vi "0516205_鍾禾翊_HW2.vi"() -> ()   [LabVIEW 2018]
panel:
  out "ByNum":dbl[](array[numeric])
  out "ByNum":dbl
  out "Slope":bool
  out "size(s)":i32[](array[numeric])
  out "Result Array":dbl[][](array[numeric])
  in  "Input N":i32=4
  out "Array 3":i32[](array[numeric])
  # "By 0"
  # "By 1"
  # "By 2"
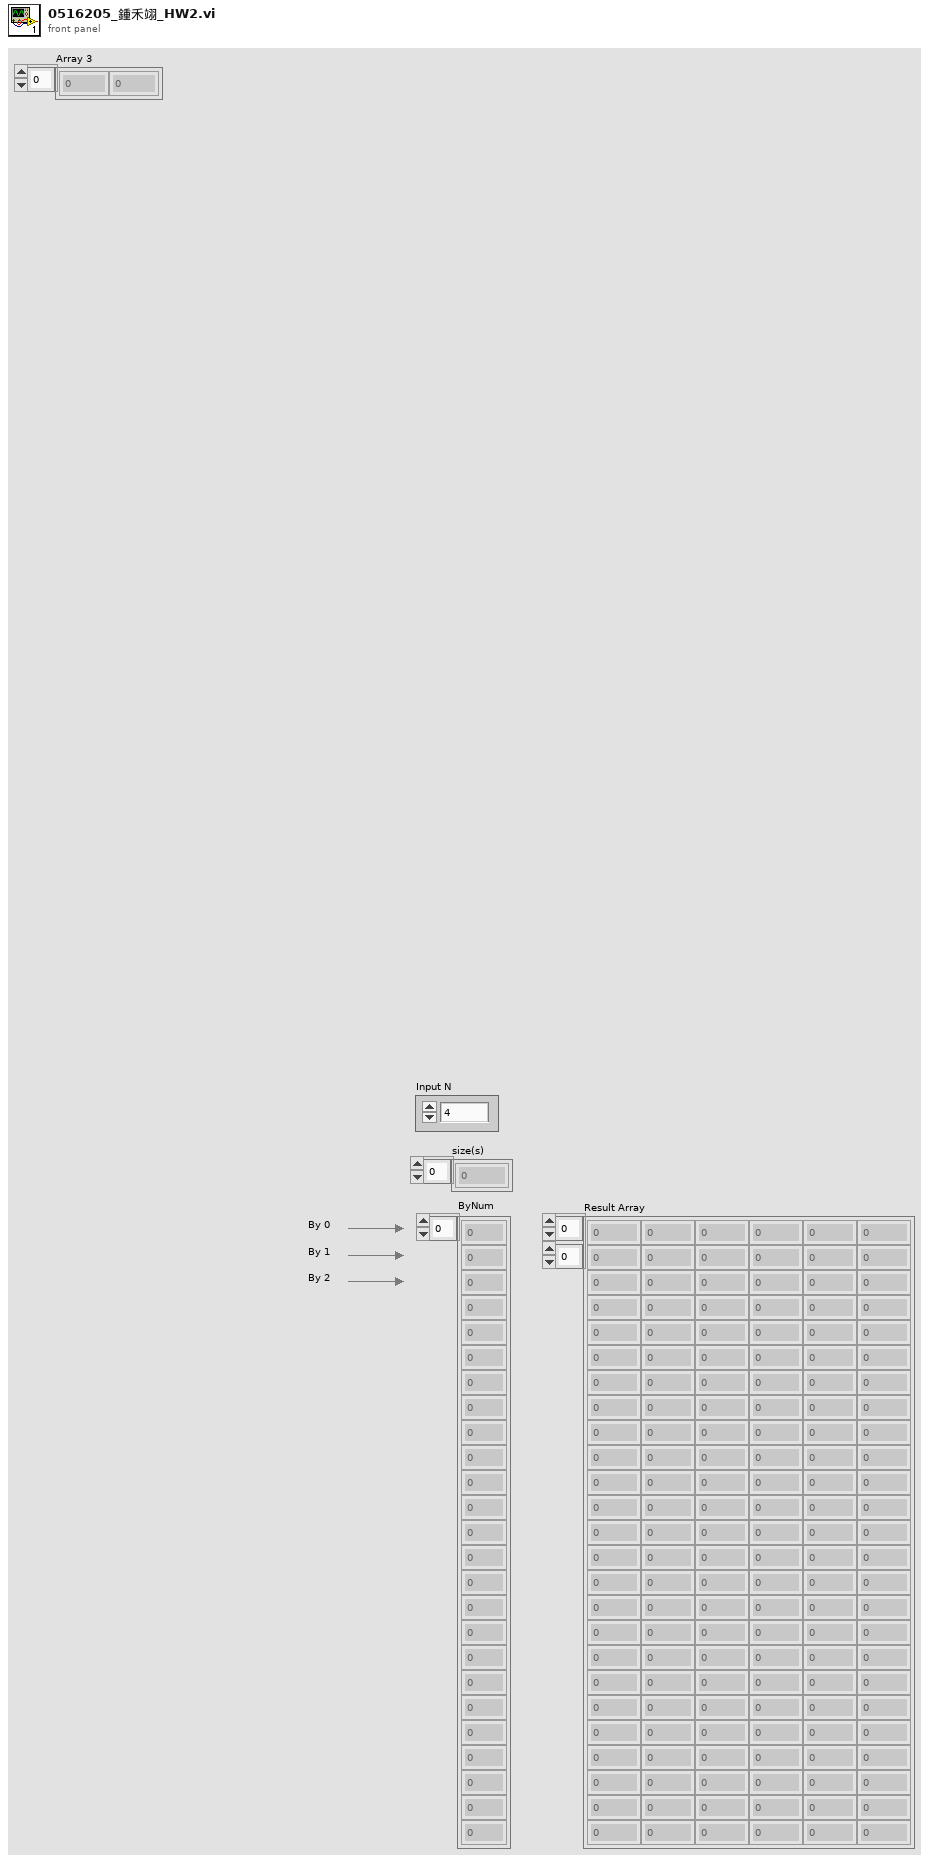
[diagram p1: front panel]
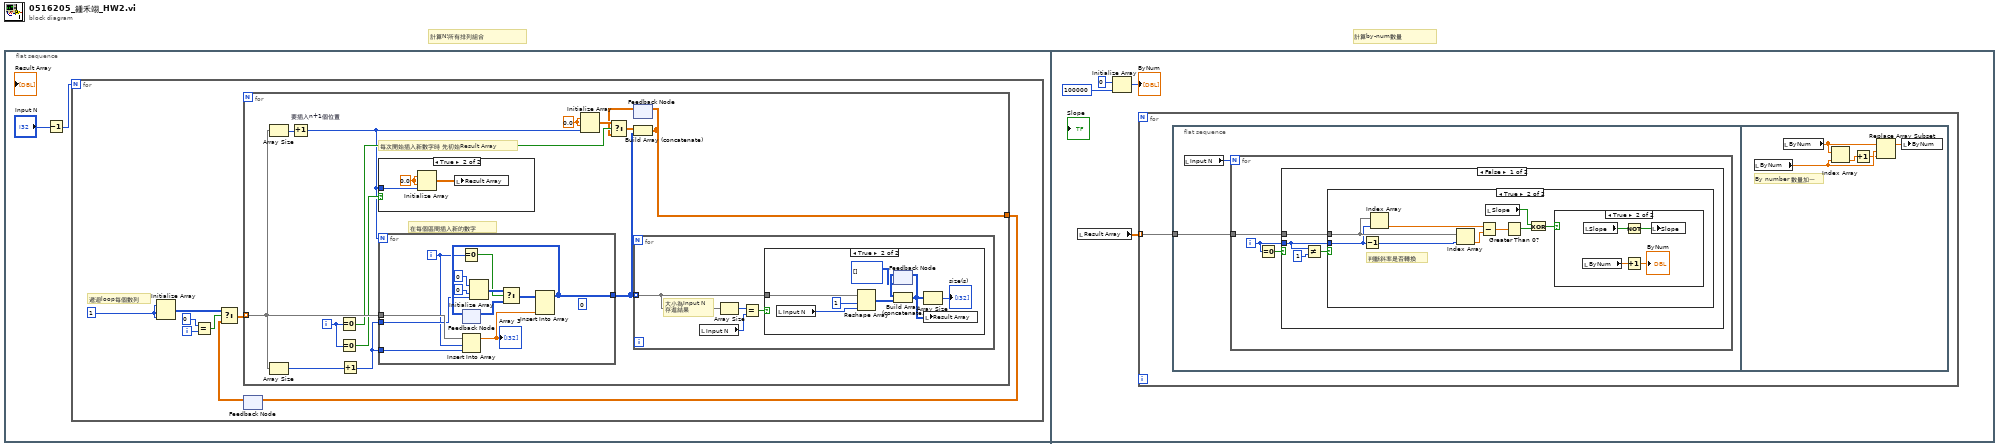
[diagram p0: block diagram]
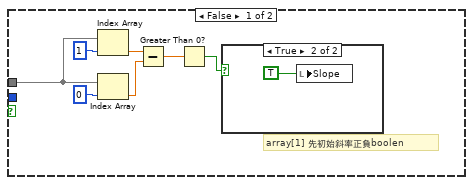
[diagram p4: hidden frame]
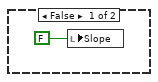
[diagram p5: hidden frame]
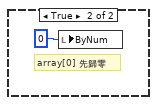
[diagram p7: hidden frame]
diagram:
  # "計算N!所有排列組合"
  # "計算by-num數量"
  n1 = flat-sequence {
    frame #0 {
      n2 = Decrement(x="Input N") -> (x-1=w1:i32)
      n3 = for {
        N: w1 -> [_]
        i -> [w5]
        w10 = 1
        # "遞迴loop每個數列"
        n4 = Initialize Array(w10, w10, w10) -> (w7:i32[][])
        n5 = Equal?(x=0, y=w5) -> (x = y?=w8:bool)
        n6 = feedback #1() -> (w3:dbl[][])  [unwired: 1 in]
        n7 = Select(t=w7, s=w8, f=w3) -> (s? t:f=w6:dbl[][])
        n8 = for {
          tunnel: [w20] -> w4
          tunnel: w6 -> [w22] mode=indexing
          i -> [w14]
          w11 = 0.0 ("element")
          # "每次開始插入新數字時 先初始Result Array"
          # "在每個區間插入新的數字"
          n9 = Array Size(array=w22) -> (size(s)=w24:i32)
          n10 = Array Size(array=w22) -> (size(s)=w23:i32)
          n11 = Increment "要插入n+1個位置"(x=w24) -> (x+1=w12:i32)
          n12 = Equal To 0?(x=w14) -> (x = 0?=w19:bool)
          n13 = Equal To 0?(x=w14) -> (x = 0?=w13:bool)
          n14 = Increment(x=w23) -> (x+1=w21:i32)
          n15 = case shown="True" w13 {
            tunnel: w12 -> [_ w25]
            frame False {
            }
            frame True {
              w27 = 0.0 ("element")
              n16 = Initialize Array(w27, w27, w25) -> (w26:dbl[][])
              n17 = local write "Result Array"(w26) -> ()
            }
          }
          n18 = for {
            N: w12 -> [_]
            tunnel: w22 -> [w50]
            tunnel: w21 -> [w43]
            tunnel: [w48] -> w15
            tunnel: w21 -> [w44]
            i -> [w40]
            (unwired) 0
            n19 = Equal To 0?(x=w40) -> (x = 0?=w41:bool)
            n20 = feedback #2() -> (w49:i32[][])  [unwired: 1 in]
            n21 = Insert Into Array(array=w50, index=w40, new element=w43) -> (w42:dbl[])
            "Array 3" <- w42
            n22 = Initialize Array(0, 0, w44) -> (w45:i32[][])
            n23 = Select(t=w45, s=w41, f=w49) -> (s? t:f=w51:i32[][])
            n24 = Insert Into Array(array=w51, new element=w42) -> (w48:i32[][])  [unwired: 2 in]
            n25 = feedback-in #2(w48) -> ()
          }
          n26 = Initialize Array(w11, w11, w12) -> (w18:dbl[][])
          n27 = feedback #3() -> (w17:dbl[][])  [unwired: 1 in]
          n28 = Select(t=w18, s=w19, f=w17) -> (s? t:f=w16:dbl[][])
          n29 = Build Array (concatenate)(w16, w15) -> (w20:dbl[][])
          n30 = feedback-in #3(w20) -> ()
          n31 = for {
            tunnel: w15 -> [w29] mode=indexing
            # "大小為Input N\n存進結果"
            n32 = local read "Input N"() -> (w28:i32)
            n33 = Array Size(array=w29) -> (size(s)=w31:i32)
            n34 = Equal?(x=w31, y=w28) -> (x = y?=w30:bool)
            n35 = case shown="True" w30 {
              tunnel: w29 -> [_ w36]
              frame False {
              }
              frame True {
                n36 = local read "Input N"() -> (w37:i32)
                n37 = Reshape Array(w36, 1, w37) -> (w38:i32[][])
                n38 = feedback #4(i32[][] []) -> (w35:i32[][])
                n39 = Build Array (concatenate)(w35, w38) -> (w34:i32[][])
                n40 = feedback-in #4(w34) -> ()
                n41 = Array Size(array=w34) -> (size(s)=→"size(s)":i32[])
                n42 = local write "Result Array"(w34) -> ()
              }
            }
          }
        }
        n43 = feedback-in #1(w4) -> ()
      }
    }
    frame #1 {
      n44 = local read "Result Array"() -> (w52:dbl[][])
      n45 = Initialize Array(0, 100000) -> (→"ByNum":i32[])
      n46 = for {
        tunnel: w52 -> [w56] mode=indexing
        n47 = flat-sequence {
          tunnel: w56 -> [w58]
          frame #0 {
            n48 = local read "Input N"() -> (w57:i32)
            n49 = for {
              N: w57 -> [_]
              tunnel: w58 -> [w61]
              i -> [w59]
              n50 = Equal To 0?(x=w59) -> (x = 0?=w60:bool)
              n51 = case shown="False" w60 {
                tunnel: w59 -> [w63 _]
                tunnel: w61 -> [w65 _]
                frame False {
                  n52 = Not Equal?(x=w63, y=1) -> (x != y?=w62:bool)
                  n53 = case shown="True" w62 {
                    tunnel: w63 -> [_ w75]
                    tunnel: w65 -> [w72 w78]
                    frame False {
                      # "array[1] 先初始斜率正負boolen"
                      n54 = Index Array(array=w72, index=1) -> (element=w69:dbl)
                      n55 = Index Array(array=w72, index=0) -> (element=w68:dbl)
                      n56 = Subtract(x=w69, y=w68) -> (x-y=w67:dbl)
                      n57 = Greater Than 0?(x=w67) -> (x > 0?=w66:bool)
                      n58 = case shown="True" w66 {
                        frame False {
                          n59 = local write "Slope"(FALSE) -> ()
                        }
                        frame True {
                          n60 = local write "Slope"(TRUE) -> ()
                        }
                      }
                    }
                    frame True {
                      # "判斷斜率是否轉換"
                      n61 = Decrement(x=w75) -> (x-1=w83:i32)
                      n62 = Index Array(array=w78, index=w75) -> (element=w76:dbl)
                      n63 = Index Array(array=w78, index=w83) -> (element=w77:dbl)
                      n64 = Subtract(x=w76, y=w77) -> (x-y=w82:dbl)
                      n65 = local read "Slope"() -> (w80:bool)
                      n66 = Greater Than 0?(x=w82) -> (x > 0?=w81:bool)
                      n67 = Exclusive Or(1:w81, 2:w80) -> (0:w79:bool)
                      n68 = case shown="True" w79 {
                        frame False {
                        }
                        frame True {
                          n69 = local read "ByNum"() -> (w85:dbl)
                          n70 = local read "Slope"() -> (w87:bool)
                          n71 = Not(x=w87) -> (.not. x?=w86:bool)
                          n72 = Increment(x=w85) -> (x+1=→"ByNum":dbl)
                          n73 = local write "Slope"(w86) -> ()
                        }
                      }
                    }
                  }
                }
                frame True {
                  # "array[0] 先歸零"
                  n74 = local write "ByNum"(0) -> ()
                }
              }
            }
          }
          frame #1 {
            # "By number 數量加一"
            n75 = local read "ByNum"() -> (w91:dbl)
            n76 = local read "ByNum"() -> (w92:dbl[])
            n77 = Index Array(array=w92, index=w91) -> (element=w93:dbl)
            n78 = Increment(x=w93) -> (x+1=w90:dbl)
            n79 = Replace Array Subset(array=w92, new element=w90, index=w91) -> (w89:dbl[])
            n80 = local write "ByNum"(w89) -> ()
          }
        }
      }
    }
  }
